vi "Read Problem.vi"(8 "error in (no error)":errorcluster, 11 "file path (use dialog)":path=path "") -> (0 "error out":errorcluster, 3 "svm_problem":T1)   [LabVIEW 2014]
doc: "Reads a file containing libsvm-formatted training data. For example from the data sets page on the official libsvm page."
uses:
  LibSVM Sparse/Wrapper API/Controls/svm_problem.ctl
  LibSVM Sparse/Wrapper API/Controls/svm_node.ctl
  <userlib>/_OpenG.lib/string/string.llb/Trim Whitespace (String)__ogtk.vi
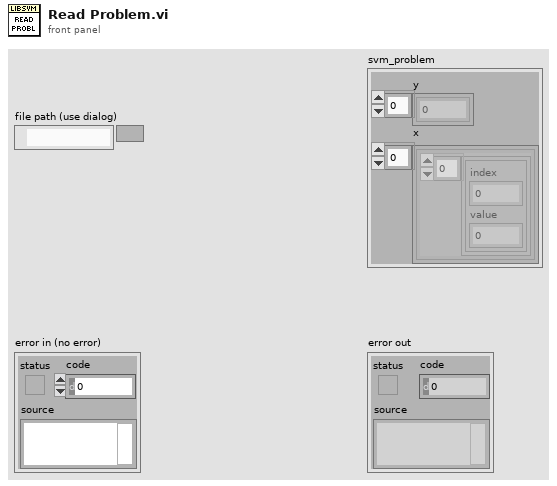
[diagram p1: front panel]
types:
  T1 = typedef "svm_problem.ctl" = cluster{"y":dbl[], "x":cluster{T2[]}[]}
  T2 = typedef "svm_node.ctl" = cluster{"index":i32, "value":dbl}
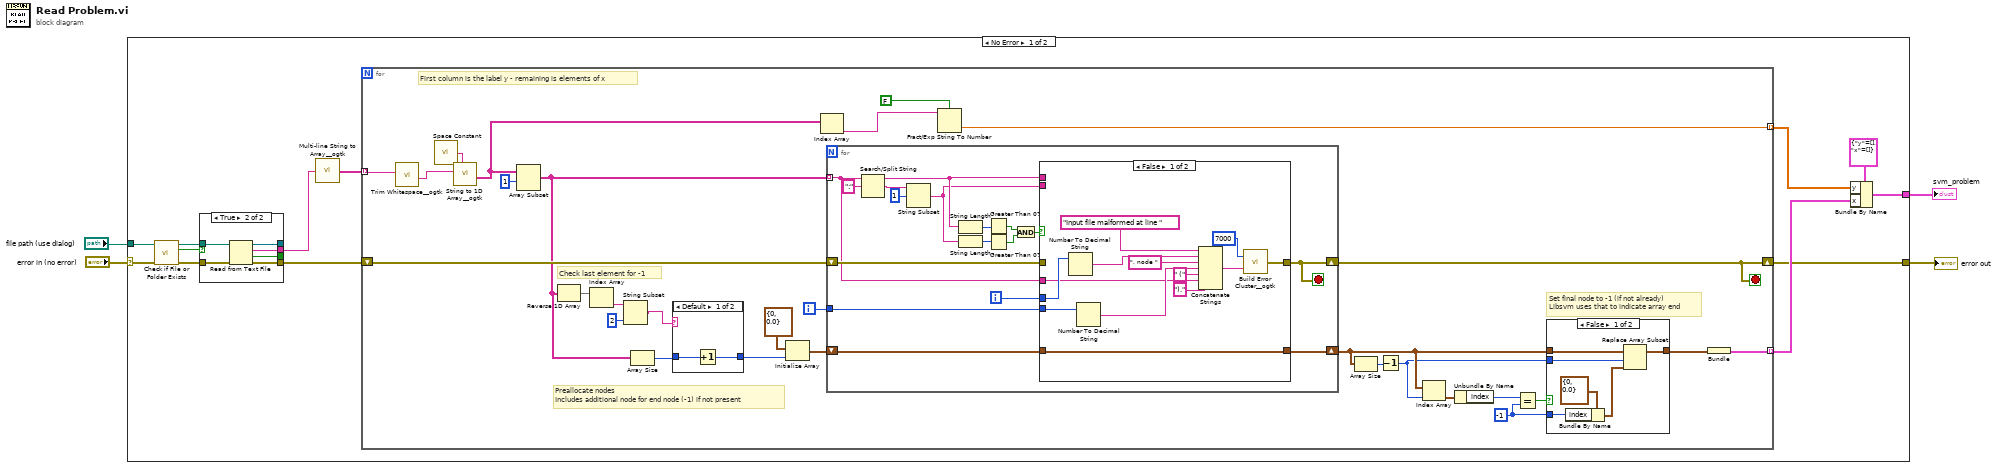
[diagram p0: block diagram]
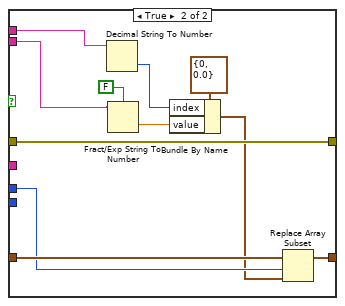
[diagram p4: hidden frame]
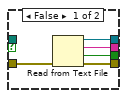
[diagram p5: hidden frame]
diagram:
  n1 = case shown="No Error" "error in (no error)" {
    selector: "error in (no error)" -> [w17 w109]
    tunnel: [w5 w109] -> w4
    tunnel: "file path (use dialog)" -> [w15 _]
    tunnel: [w6 _] -> w1
    frame No Error {
      n2 = call <vilib>:"Check if File or Folder Exists.vi"("error in (no error)"=w17, "path"=w15) -> ("error out"=w16:errorcluster, "file or folder exists?"=w14:bool, "dup path"=w13:path)  [unwired: 7 in]
      n3 = case shown="True" w14 {
        tunnel: w16 -> [w102 w108]
        tunnel: w13 -> [_ w106]
        tunnel: [w101 w107] -> w11
        tunnel: [w100 w105] -> _
        tunnel: [w99 w104] -> _
        tunnel: [w98 w103] -> w12
        frame False {
          n4 = Read from Text File(error in=w102) -> (refnum out=w100:refnum<file>, text=w98:string, cancelled=w99:bool, error out=w101:errorcluster)  [unwired: 3 in]
        }
        frame True {
          n5 = Read from Text File(file (use dialog)=w106, error in=w108) -> (refnum out=w105:refnum<file>, text=w103:string, cancelled=w104:bool, error out=w107:errorcluster)  [unwired: 2 in]
        }
      }
      n6 = call <userlib>:"Multi-line String to Array__ogtk.vi"("string"=w12) -> ("lines"=w10:string[])
      n7 = for {
        tunnel: w10 -> [w19] mode=indexing
        tunnel: [w43] -> w7 mode=indexing
        tunnel: [w40] -> w8 mode=indexing
        shift-right: [w39] -> w5
        shift-left: w11 -> [w42]
        i -> [w41]
        stop <- w39 stop-if-true
        w27 = -1 ("y")
        # "Check last element for -1"
        # "Set final node to -1 (if not already)\nLibsvm uses that to indicate array end"
        # "Preallocate nodes\nIncludes additional node for end node (-1) if not present"
        # "First column is the label y - remaining is elements of x"
        n8 = call-poly <userlib>:"Trim Whitespace__ogtk.vi"("String in"=w19) -> ("String out"=w18:string)  [unwired: 6 in]
        n9 = call <vilib>:"Space Constant.vi"() -> ("String"=w46:string)
        n10 = call <userlib>:"String to 1D Array__ogtk.vi"("delimiter (Tab)"=w46, "string"=w18) -> ("Array of Strings"=w37:string[])  [unwired: 9 in]
        n11 = Array Subset(array=w37, index=1) -> (w20:string[])  [unwired: 1 in]
        n12 = Reverse 1D Array(array=w20) -> (reversed array=w26:string[])
        n13 = Index Array(array=w26) -> (element=w25:string)  [unwired: 1 in]
        n14 = String Subset(string=w25, length (rest)=2 ("length (rest)")) -> (substring=w23:string)  [unwired: 1 in]
        n15 = Array Size(array=w20) -> (size(s)=w22:i32)
        n16 = case shown="Default" w23 {
          tunnel: w22 -> [w47 w49]
          tunnel: [w48 w49] -> w21
          frame Default {
            n17 = Increment(x=w47) -> (x+1=w48:i32)
          }
          frame "-1" {
          }
        }
        n18 = Initialize Array(T2 {"index"=0, "value"=0.0} ("svm_node"), w21) -> (w35:T2[])
        n19 = Index Array(array=w37) -> (element=w45:string)  [unwired: 1 in]
        n20 = for {
          tunnel: w20 -> [w66] mode=indexing
          tunnel: w41 -> [w58]
          shift-right: [w63] -> w39
          shift-left: w42 -> [w68]
          shift-right: [w64] -> w32
          shift-left: w35 -> [w57]
          i -> [w67]
          stop <- w63 stop-if-true
          n21 = Search/Split String(string=w66, search string/char (-)=":") -> (substring before match=w65:string, match + rest of string=w61:string)  [unwired: 1 in, 1 out]
          n22 = String Subset(string=w61, offset (0)=1) -> (substring=w59:string)  [unwired: 1 in]
          n23 = String Length(string=w65) -> (length=w62:i32)
          n24 = String Length(string=w59) -> (length=w72:i32)
          n25 = Greater Than 0?(x=w62) -> (x > 0?=w71:bool)
          n26 = Greater Than 0?(x=w72) -> (x > 0?=w70:bool)
          n27 = And(x=w71, y=w70) -> (x .and. y?=w69:bool)
          n28 = case shown="False" w69 {
            tunnel: w68 -> [_ w97]
            tunnel: [w85 w97] -> w63
            tunnel: w67 -> [w84 w91]
            tunnel: w58 -> [w83 _]
            tunnel: w66 -> [w76 _]
            tunnel: w65 -> [_ w95]
            tunnel: w59 -> [_ w94]
            tunnel: [w74 w93] -> w64
            tunnel: w57 -> [w74 w92]
            frame False {
              n29 = Number To Decimal String(number=w84) -> (decimal integer string=w81:string)  [unwired: 1 in]
              n30 = Number To Decimal String(number=w83) -> (decimal integer string=w79:string)  [unwired: 1 in]
              n31 = Concatenate Strings("Input file malformed at line " ("String to Prepend to source (\"\")"), w81, ", node " ("string"), w79, " (" ("string"), w76, ")." ("string")) -> (w75:string)
              n32 = call <userlib>:"Build Error Cluster__ogtk.vi"("String to Prepend to source (\"\")"=w75, "code"=7000) -> ("error out"=w85:errorcluster)
            }
            frame True {
              n33 = Decimal String To Number(string=w95) -> (number=w87:i32)  [unwired: 2 in, 1 out]
              n34 = Fract/Exp String To Number(use system decimal point (T)=FALSE, string=w94) -> (number=w88:dbl)  [unwired: 2 in, 1 out]
              n35 = Bundle By Name(cluster=T2 {"index"=0, "value"=0.0} ("svm_node"), "index"=w87, "value"=w88) -> (w89:T2)
              n36 = Replace Array Subset(array=w92, new element=w89, index=w91) -> (w93:T2[])
            }
          }
        }
        n37 = Fract/Exp String To Number(use system decimal point (T)=FALSE, string=w45) -> (number=w43:dbl)  [unwired: 2 in, 1 out]
        n38 = Array Size(array=w32) -> (size(s)=w33:i32)
        n39 = Decrement(x=w33) -> (x-1=w28:i32)
        n40 = Index Array(array=w32, index=w28) -> (element=w31:T2)
        n41 = Unbundle By Name(w31) -> ("index"=w30:i32)
        n42 = Equal?(x=w30, y=w27) -> (x = y?=w29:bool)
        n43 = case shown="False" w29 {
          tunnel: [w55 w56] -> w34
          tunnel: w32 -> [w54 w56]
          tunnel: w28 -> [w53 _]
          tunnel: w27 -> [w51 _]
          frame False {
            n44 = Bundle By Name(cluster=T2 {"index"=0, "value"=0.0} ("svm_node"), "index"=w51) -> (w50:T2)
            n45 = Replace Array Subset(array=w54, new element=w50, index=w53) -> (w55:T2[])
          }
          frame True {
          }
        }
        n46 = Bundle(w34) -> (w40:cluster{T2[]})  [unwired: 1 in]
      }
      n47 = Bundle By Name(cluster=T1 {"y"=[], "x"=[]} ("svm_problem"), "y"=w7, "x"=w8) -> (w6:T1)
    }
    frame Error {
    }
  }
  "error out" <- w4
  "svm_problem" <- w1
